vi "ReadTileFromPNG.vi"(8 "error in (no error)":errorcluster, 11 "path to PNG file":path=path "/home/lvuser/natinst/bin/data/Aesomatica_16x16.png") -> (0 "error out":errorcluster, 3 "TileBufferData":fxp<+,3,3>[](array[numeric]))   [LabVIEW 2019, in "RT_Game.lvlib" / "Game.lvclass"]
uses:
  Game.lvclass
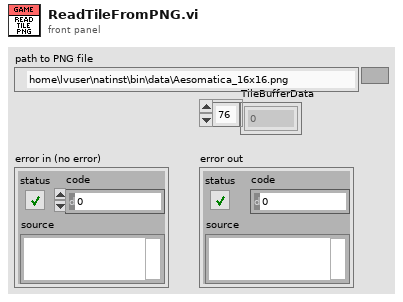
[diagram p1: front panel]
types:
  T1 = typedef "Color (U64)" = cluster{"Plane 3 (Blue)":u16, "Plane 2 (Green)":u16, "Plane 1 (Red)":u16, "Plane 4 (alpha)":u16}
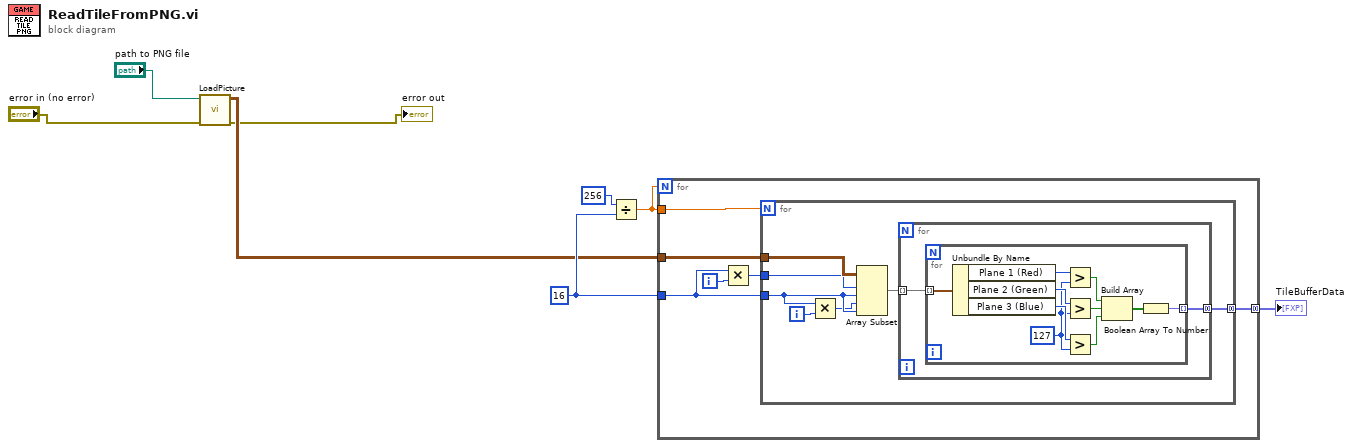
[diagram p0: block diagram]
diagram:
  w5 = 16 ("length")
  n1 = call "LoadPicture.vi"("error in (no error)"="error in (no error)", "path to PNG file"="path to PNG file") -> ("error out"=→"error out":errorcluster, "Image Pixels (U64)"=w2:T1[][])  [unwired: 8 in]
  n2 = Divide(x=256 ("length"), y=w5) -> (x/y=w6:dbl)
  n3 = for {
    N: w6 -> [_]
    tunnel: w2 -> [w14]
    tunnel: w5 -> [w11]
    tunnel: [w13] -> w7 mode=concatenating
    tunnel: w6 -> [w9]
    i -> [w12]
    n4 = Multiply(x=w11, y=w12) -> (x*y=w10:i32)
    n5 = for {
      N: w9 -> [_]
      tunnel: w14 -> [w21]
      tunnel: w11 -> [w19]
      tunnel: [w18] -> w13 mode=concatenating
      tunnel: w10 -> [w15]
      i -> [w20]
      n6 = Multiply(x=w19, y=w20) -> (x*y=w16:i32)
      n7 = Array Subset(array=w21, index (row)=w15, length (row)=w19, index (col)=w16, length (col)=w19) -> (w17:T1[][])
      n8 = for {
        tunnel: w17 -> [w23] mode=indexing
        tunnel: [w22] -> w18 mode=concatenating
        n9 = for {
          tunnel: w23 -> [w33] mode=indexing
          tunnel: [w27] -> w22 mode=indexing
          w29 = u8 127 ("y")
          n10 = Unbundle By Name(w33) -> ("Plane 1 (Red)"=w32:u16, "Plane 2 (Green)"=w31:u16, "Plane 3 (Blue)"=w30:u16)
          n11 = Greater?(x=w32, y=w29) -> (0:w26:bool)
          n12 = Greater?(x=w31, y=w29) -> (0:w25:bool)
          n13 = Greater?(x=w30, y=w29) -> (0:w24:bool)
          n14 = Build Array(w26, w25, w24) -> (w28:bool[])
          n15 = Boolean Array To Number(Boolean array=w28) -> (number=w27:fxp<+,3,3>)
        }
      }
    }
  }
  "TileBufferData" <- w7
